vi "PV Fehler.vi"(8 "error in (no error)":errorcluster caption="Fehler (Eingang, kein Fehler)", 10 "Istwerte":u16[](array[numeric]), 11 "Steuerung PNS Eingang":refnum<class "Steuerung PNS.lvclass">) -> (0 "error out":errorcluster caption="Fehler (Ausgang)", 3 "Steuerung PNS Ausgang":refnum<class "Steuerung PNS.lvclass">)   [LabVIEW 2020, in "Steuerung PNS.lvclass"]
doc: "Error Code für PNS setzen.\nRIW"
uses:
  Steuerung PNS.lvclass
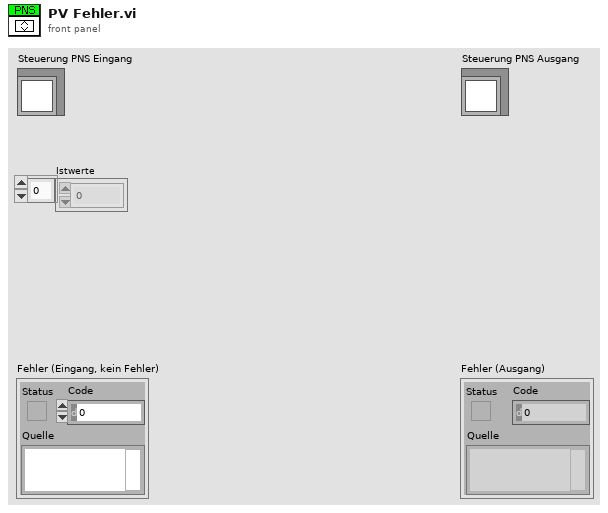
[diagram p1: front panel]
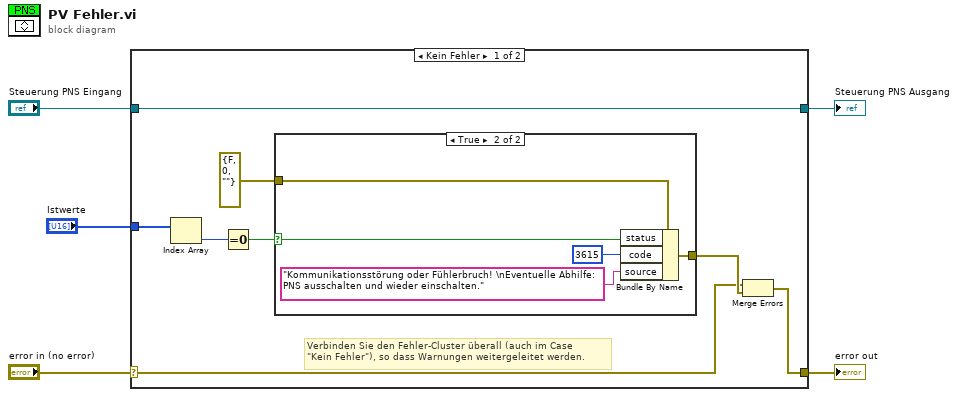
[diagram p0: block diagram]
diagram:
  n1 = case shown="Kein Fehler" "error in (no error)" {
    selector: "error in (no error)" -> [w7 w21]
    tunnel: [w6 w21] -> w4
    tunnel: [w13 w20] -> w2
    tunnel: "Steuerung PNS Eingang" -> [w13 w20]
    tunnel: "Istwerte" -> [w11 _]
    frame No Error {
      # "Verbinden Sie den Fehler-Cluster überall (auch im Case\n\"Kein Fehler\"), so dass Warnungen weitergeleitet werden."
      n2 = Index Array(array=w11) -> (element=w12:u16)  [unwired: 1 in]
      n3 = Equal To 0?(x=w12) -> (x = 0?=w10:bool)
      n4 = case shown="True" w10 {
        selector: w10 -> [_ w15]
        tunnel: errorcluster {"status"=FALSE, "code"=0, "source"=""} ("error out") -> [w14 w19]
        tunnel: [w14 w16] -> w8
        frame False {
        }
        frame True {
          n5 = Bundle By Name(cluster=w19, "status"=w15, "code"=3615, "source"="Kommunikationsstörung oder Fühlerbruch! \nEventuelle Abhilfe: PNS ausschalten und wieder einschalten.") -> (w16:errorcluster)
        }
      }
      n6 = Merge Errors(w7, w8) -> (w6:errorcluster)
    }
    frame Error {
    }
  }
  "error out" <- w4
  "Steuerung PNS Ausgang" <- w2
